vi "OneButtonDialogAsynch.vi"(8 "error in (no error)":errorcluster, 11 "Message to Display":string) -> (0 "error out":errorcluster)   [LabVIEW 2013]
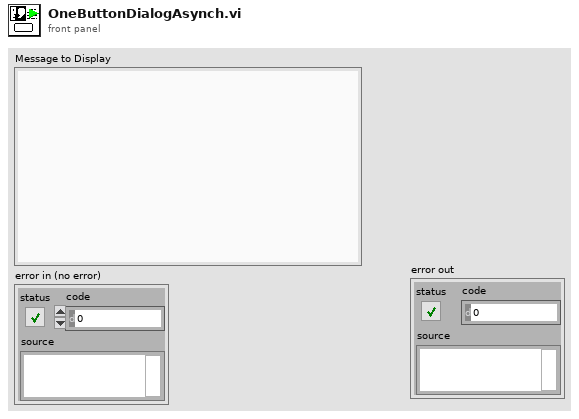
[diagram p1: front panel]
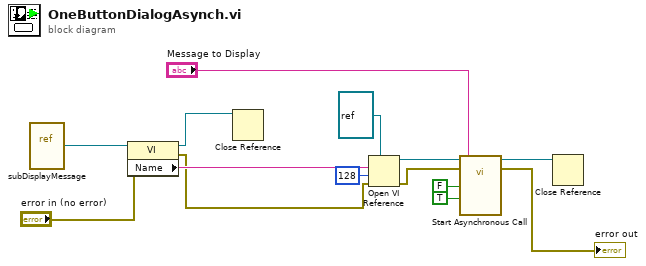
[diagram p0: block diagram]
diagram:
  n1 = vi-ref <vilib>:"subDisplayMessage.vi"() -> (w13:refnum<vi>)
  n2 = property class="VI"(reference=w13, error in="error in (no error)") -> (reference out=w9:refnum<vi>, error out=w4:errorcluster, "Name"=w12:string)
  n3 = Close Reference(reference=w9) -> ()  [unwired: 1 in, 1 out]
  n4 = Open VI Reference(type specifier VI Refnum (for type only)=refnum<vi> refnum, vi path=w12, options=128, error in (no error)=w4) -> (vi reference=w10:refnum<vi>, error out=w3:errorcluster)  [unwired: 2 in]
  n5 = call-by-ref "Start Asynchronous Call"(reference=w10, error in=w3, "Enable Message"=TRUE, "Show 'Cancel' Button"=FALSE, "Message to Display"="Message to Display") -> (reference out=w8:refnum<vi>, error out=→"error out":errorcluster)  [unwired: 7 in, 2 out]
  n6 = Close Reference(reference=w8) -> ()  [unwired: 1 in, 1 out]
